vi "DCAM_example_multifunc_scmos_frame_acquisition.vi"() -> ()   [LabVIEW 2015]
uses:
  <vilib>/Utility/miscctls.llb/LVRectTypeDef.ctl
panel:
  out "Image":u16[][](graph)
  in  "Stop Button":bool
  in  "Acquire Frames Button":bool
  in  "Take Snapshot Button":bool
  in  "Preview Mode Button":bool
  out "Start Trigger Mode":string
  out "error out":errorcluster
  out "Plot Area Bounds":T1
  in  "Exposure":dbl min=0.0010036691729323308 max=10.000004210526315 step=1e-08
  in  "Scan Mode":dbl min=1.0 max=2.0 step=1.0
  in  "Binning":u16(ring) items=["1x1"=1, "2x2"=2, "4x4"=4]
  out "Exposure":dbl
  out "Scan Mode":dbl
  out "S Vert Width":i32
  out "S Horiz Width":i32
  out "S Vert Offset":i32
  out "S Horiz Offset":i32
  in  "Vertical Width":i32 min=4 max=2048 step=4
  in  "Vertical Offset":i32 min=0 max=0 step=4
  in  "Horizontal Width":i32 min=4 max=2048 step=4
  in  "Horizontal Offset":i32 min=0 max=0 step=4
  in  "Number of Frames":dbl
  out "Timeseries Save Path":path
  out "Snapshot Save Path":path
  out "Timeseries Base Filename":string
  out "Snapshot Base Filename":string
  in  "Timeseries Base Filename":string
  in  "Timeseries Save Path":path
  in  "Snapshot Base Filename":string
  in  "Save Snapshots":bool caption="Save Snapshot"
  in  "Snapshot Save Path":path
  in  "Start Trigger Mode":u32(ring)=1 items=["Internal"=1, "External Edge"=2, "External Level"=4, "Software"=32, "Fast Repetition"=64, "TDI"=128, "Trigger Start"=512, "Sync Readout"=1024]
  out "Model":string
  out "Camera ID":string
  out "Firmware":string
  out "DCAM Ver.":string
  out "Library Ver.":string
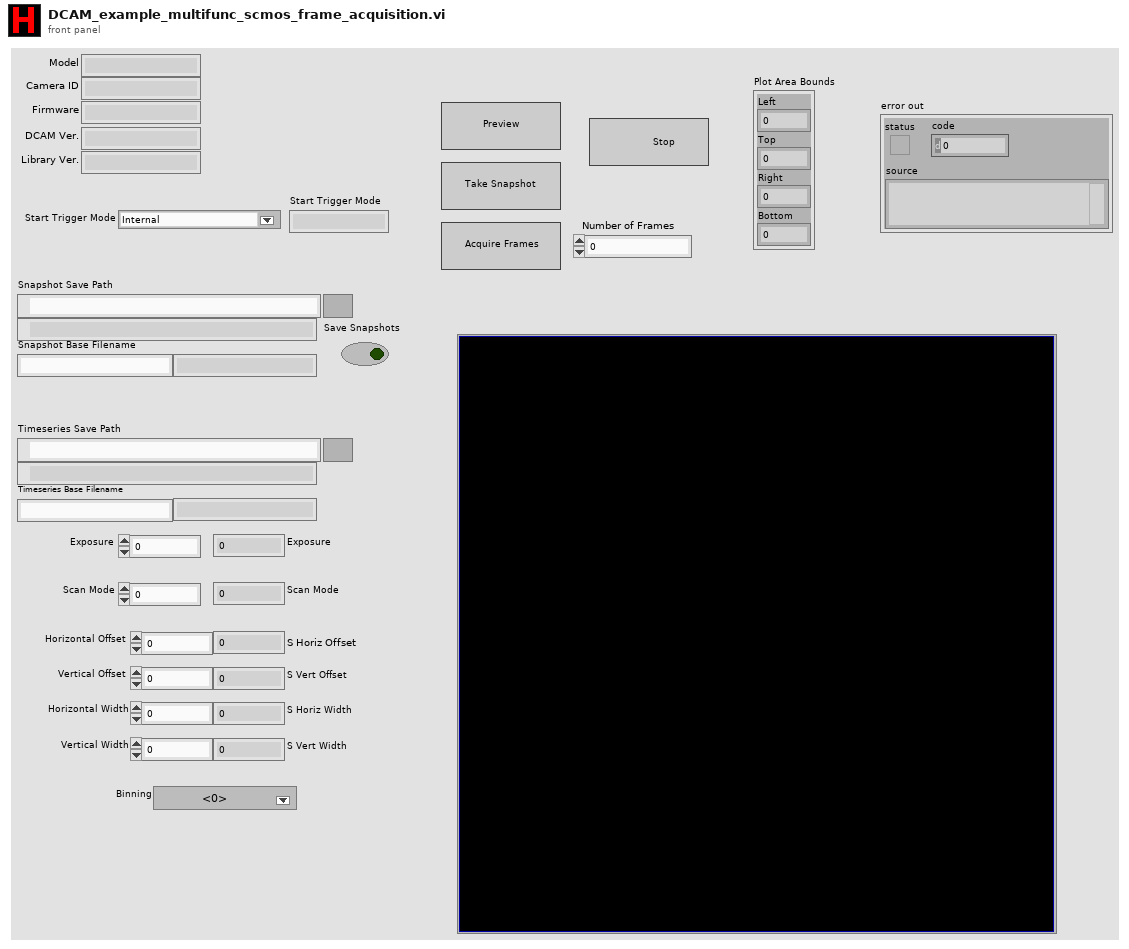
[diagram p1: front panel]
types:
  T1 = typedef "LVRectTypeDef.ctl" = cluster{"Left":i16, "Top":i16, "Right":i16, "Bottom":i16}
  T2 = cluster{"Capture Library":string, "DCAM-API":string}
  T3 = cluster{"Mode":u32, "Polarity":u16, "Times":u32, "Delay":dbl}
  T4 = cluster{"Mode":u32, "Polarity":u32, "Period":dbl, "Delay":dbl}
  T5 = cluster{"Model":string, "Camera ID":string, "Firmware":string}
  T6 = cluster{"Value":i32, "Minimum":i32, "Maximum":i32, "Increment":i32}
  T7 = cluster{"height":u32, "width":u32, "datatype":u32}
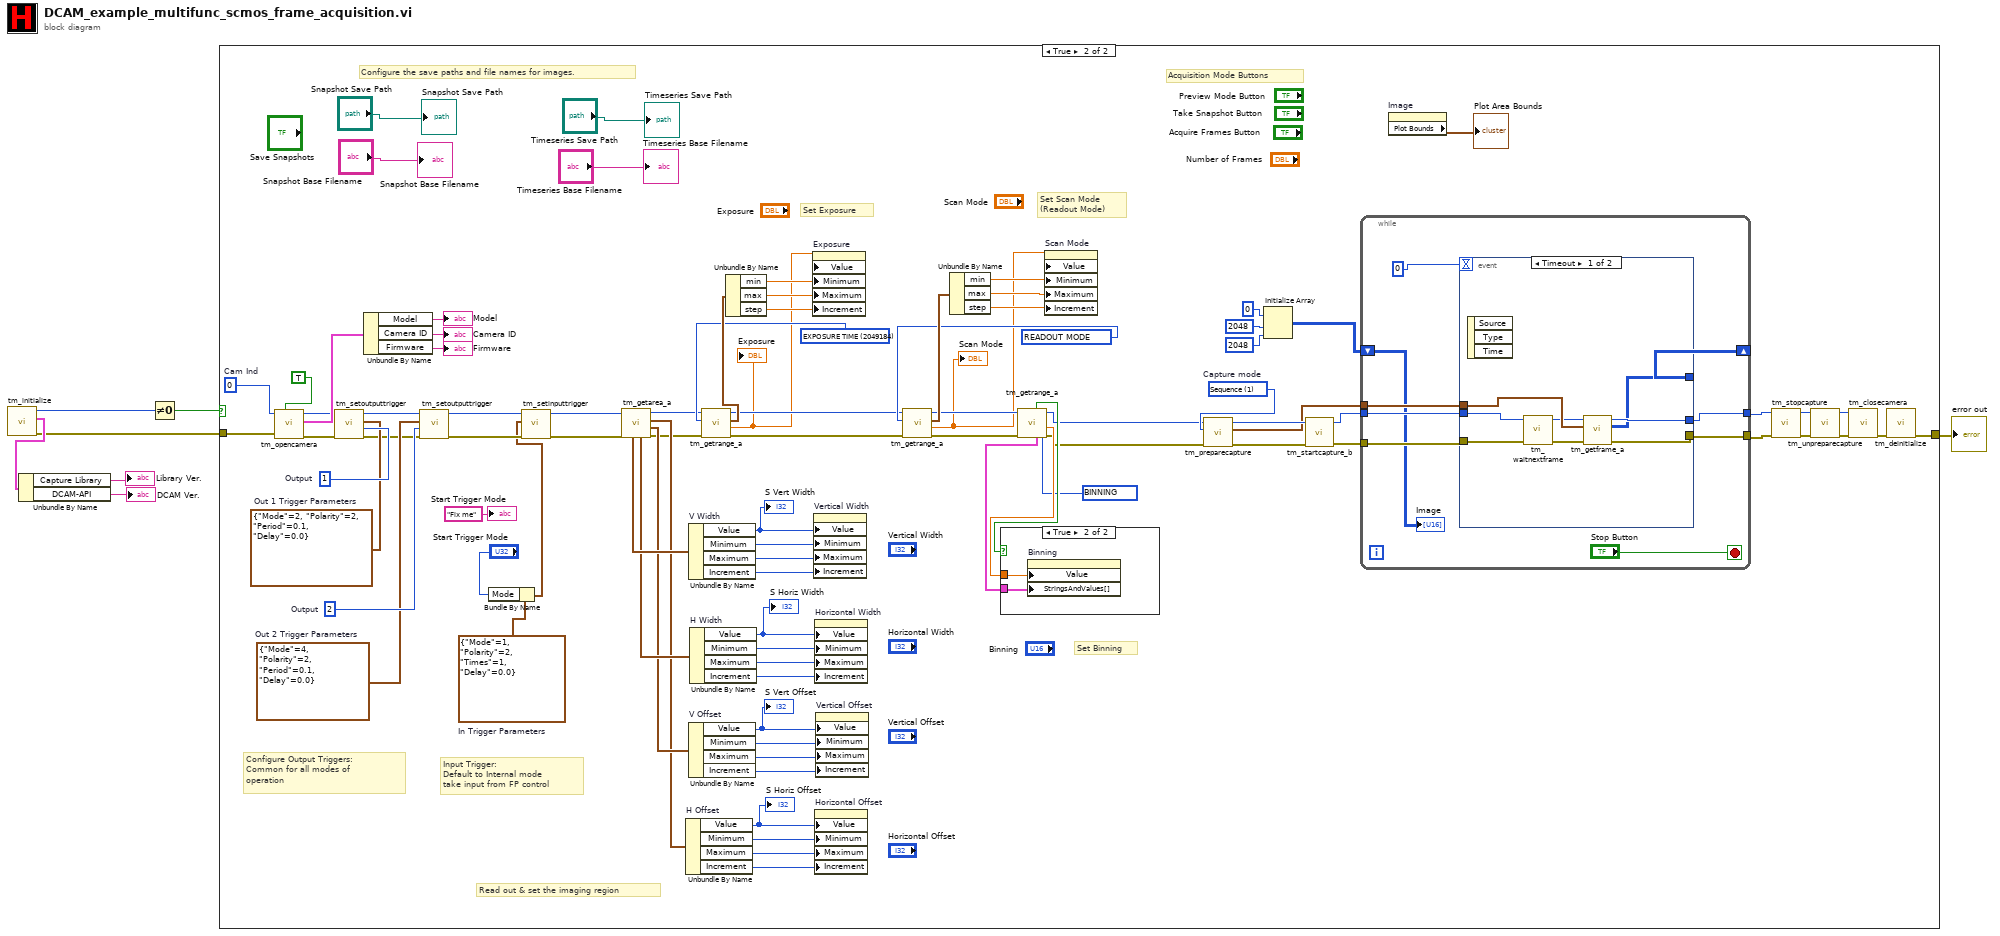
[diagram p0: block diagram]
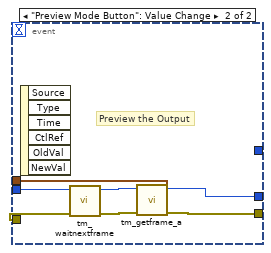
[diagram p3: hidden frame]
diagram:
  n1 = call <userlib>:"tm_initialize.vi"() -> ("error out"=w3:errorcluster, "Version Info"=w4:T2, "Number Of Cameras"=w7:u32)  [unwired: 8 in, 1 out]
  n2 = Unbundle By Name(w4) -> ("Capture Library"=→"Library Ver.":string, "DCAM-API"=→"DCAM Ver.":string)
  n3 = Not Equal To 0?(x=w7) -> (x != 0?=w2:bool)
  n4 = case shown="True" w2 {
    tunnel: w3 -> [w8 w85]
    tunnel: [w8 w37] -> w1
    frame False {
    }
    frame True {
      w20 = 1 items=["Snap", "Sequence"]  # Capture mode
      w47 = u32 2049184 items=["BINNING"=4215968, "BITS PER CHANNEL"=4342976, "ACTIVE VIEW INDEX"=4343136, "CCD MODE"=4212384, "SENSOR MODE"=4212128, "READOUT MODE"=4211872, "EXPOSURE TIME"=2049184, "CONTRAST GAIN"=3163312, "CONTRAST OFFSET"=3163328, "LIGHT MODE"=2114720, "SENSITIVITY"=2114992, "WHITE BALANCE"=3163568, "PHOTON IMAGING MODE"=2115200, "HIGH DYNAMIC RANGE MODE"=3163360, "TRIGGER SOURCE"=1066144, "TRIGGER ACTIVE"=1066160, "TRIGGER MODE"=1066400, "TRIGGER POLARITY"=1066416, "TRIGGER GLOBAL EXPOSURE"=2049680, "FIRST TRIGGER BEHAVIOR"=2049696, "TRIGGER TIMES"=1066448, "OUTPUT TRIGGER POLARITY"=1852592, "OUTPUT TRIGGER DELAY"=1852624, "OUTPUT TRIGGER PERIOD"=1852640, "TEMPERATURE"=2115232, "TEMPERATURE TARGET"=2115264, "SENSOR COOLER FAN"=2115296, "MECHANICAL SHUTTER"=2115488, "BACK FOCUS POSITION"=8422304, "FRAMEBUNDLE MODE"=4346784, "FRAMEBUNDLE NUMBER"=4346800, "LINEBUNDLE HEIGHT"=4212192, "TRIGGER CONNECTOR"=1066432, "IMAGE PIXEL TYPE"=4343296, "OUTPUT TRIGGER KIND"=1852656, "READOUT DIRECTION"=4211904, "CHANNEL SYNC"=1852352] ("Parameter")
      w48 = u32 4211872 items=["BINNING"=4215968, "BITS PER CHANNEL"=4342976, "ACTIVE VIEW INDEX"=4343136, "CCD MODE"=4212384, "SENSOR MODE"=4212128, "READOUT MODE"=4211872, "EXPOSURE TIME"=2049184, "CONTRAST GAIN"=3163312, "CONTRAST OFFSET"=3163328, "LIGHT MODE"=2114720, "SENSITIVITY"=2114992, "WHITE BALANCE"=3163568, "PHOTON IMAGING MODE"=2115200, "HIGH DYNAMIC RANGE MODE"=3163360, "TRIGGER SOURCE"=1066144, "TRIGGER ACTIVE"=1066160, "TRIGGER MODE"=1066400, "TRIGGER POLARITY"=1066416, "TRIGGER GLOBAL EXPOSURE"=2049680, "FIRST TRIGGER BEHAVIOR"=2049696, "TRIGGER TIMES"=1066448, "OUTPUT TRIGGER POLARITY"=1852592, "OUTPUT TRIGGER DELAY"=1852624, "OUTPUT TRIGGER PERIOD"=1852640, "TEMPERATURE"=2115232, "TEMPERATURE TARGET"=2115264, "SENSOR COOLER FAN"=2115296, "MECHANICAL SHUTTER"=2115488, "BACK FOCUS POSITION"=8422304, "FRAMEBUNDLE MODE"=4346784, "FRAMEBUNDLE NUMBER"=4346800, "LINEBUNDLE HEIGHT"=4212192, "TRIGGER CONNECTOR"=1066432, "IMAGE PIXEL TYPE"=4343296, "OUTPUT TRIGGER KIND"=1852656, "READOUT DIRECTION"=4211904, "CHANNEL SYNC"=1852352] ("Parameter")
      w49 = u32 4215968 items=["BINNING"=4215968, "BITS PER CHANNEL"=4342976, "ACTIVE VIEW INDEX"=4343136, "CCD MODE"=4212384, "SENSOR MODE"=4212128, "READOUT MODE"=4211872, "EXPOSURE TIME"=2049184, "CONTRAST GAIN"=3163312, "CONTRAST OFFSET"=3163328, "LIGHT MODE"=2114720, "SENSITIVITY"=2114992, "WHITE BALANCE"=3163568, "PHOTON IMAGING MODE"=2115200, "HIGH DYNAMIC RANGE MODE"=3163360, "TRIGGER SOURCE"=1066144, "TRIGGER ACTIVE"=1066160, "TRIGGER MODE"=1066400, "TRIGGER POLARITY"=1066416, "TRIGGER GLOBAL EXPOSURE"=2049680, "FIRST TRIGGER BEHAVIOR"=2049696, "TRIGGER TIMES"=1066448, "OUTPUT TRIGGER POLARITY"=1852592, "OUTPUT TRIGGER DELAY"=1852624, "OUTPUT TRIGGER PERIOD"=1852640, "TEMPERATURE"=2115232, "TEMPERATURE TARGET"=2115264, "SENSOR COOLER FAN"=2115296, "MECHANICAL SHUTTER"=2115488, "BACK FOCUS POSITION"=8422304, "FRAMEBUNDLE MODE"=4346784, "FRAMEBUNDLE NUMBER"=4346800, "LINEBUNDLE HEIGHT"=4212192, "TRIGGER CONNECTOR"=1066432, "IMAGE PIXEL TYPE"=4343296, "OUTPUT TRIGGER KIND"=1852656, "READOUT DIRECTION"=4211904, "CHANNEL SYNC"=1852352] ("Parameter")
      w80 = T3 {"Mode"=1, "Polarity"=2, "Times"=1, "Delay"=0.0}  # In Trigger Parameters
      w86 = T4 {"Mode"=4, "Polarity"=2, "Period"=0.1, "Delay"=0.0}  # Out 2 Trigger Parameters
      w87 = T4 {"Mode"=2, "Polarity"=2, "Period"=0.1, "Delay"=0.0}  # Out 1 Trigger Parameters
      w89 = 2  # Output
      w91 = 1  # Output
      w97 = 0  # Cam Ind
      # "Acquisition Mode Buttons"
      # "Configure the save paths and file names for images."
      # "Set Binning"
      # "Set Scan Mode \n(Readout Mode)"
      # "Set Exposure"
      # "Read out & set the imaging region"
      # "Input Trigger:\nDefault to Internal mode\ntake input from FP control"
      # "Configure Output Triggers: \nCommon for all modes of operation"
      n5 = call <userlib>:"tm_opencamera.vi"("Force Open"=TRUE, "error in (no error)"=w85, "Camera Index"=w97) -> ("error out"=w84:errorcluster, "Camera Details"=w96:T5, "Handle out"=w92:u32)  [unwired: 6 in]
      n6 = call <userlib>:"tm_setoutputtrigger.vi"("error in (no error)"=w84, "Index"=w91, "Parameters"=w87) -> ("error out"=w83:errorcluster, "Handle out"=w90:u32)  [unwired: 7 in]
      n7 = Unbundle By Name(w96) -> ("Model"=→"Model":string, "Camera ID"=→"Camera ID":string, "Firmware"=→"Firmware":string)
      n8 = call <userlib>:"tm_setoutputtrigger.vi"("error in (no error)"=w83, "Index"=w89, "Parameters"=w86, "Handle in"=w90) -> ("error out"=w82:errorcluster)  [unwired: 6 in, 1 out]
      n9 = Bundle By Name(cluster=w80, "Mode"="Start Trigger Mode") -> (w81:T3)
      n10 = call <userlib>:"tm_setinputtrigger.vi"("error in (no error)"=w82, "Parameters"=w81, "Handle in"=w92) -> ("error out"=w77:errorcluster, "Handle out"=w78:u32)  [unwired: 7 in]
      n11 = call <userlib>:"tm_getarea_a.vi"("error in (no error)"=w77, "Handle in"=w78) -> ("error out"=w46:errorcluster, "V Offset"=w74:T6, "H Offset"=w73:T6, "Handle out"=w45:u32, "H Width"=w75:T6, "V Width"=w76:T6)  [unwired: 4 in]
      n12 = Unbundle By Name "H Offset"(w73) -> ("Value"=w60:i32, "Minimum"=w59:i32, "Maximum"=w58:i32, "Increment"=w57:i32)
      "S Horiz Offset" <- w60
      n13 = Unbundle By Name "V Width"(w76) -> ("Value"=w72:i32, "Minimum"=w71:i32, "Maximum"=w70:i32, "Increment"=w69:i32)
      "S Vert Width" <- w72
      n14 = Unbundle By Name "V Offset"(w74) -> ("Value"=w64:i32, "Minimum"=w63:i32, "Maximum"=w62:i32, "Increment"=w61:i32)
      "S Vert Offset" <- w64
      n15 = Unbundle By Name "H Width"(w75) -> ("Value"=w68:i32, "Minimum"=w67:i32, "Maximum"=w66:i32, "Increment"=w65:i32)
      "S Horiz Width" <- w68
      n16 = call <userlib>:"tm_getrange_a.vi"("error in (no error)"=w46, "Parameter"=w47, "Handle in"=w45) -> ("error out"=w55:errorcluster, "default"=w31:dbl, "Range"=w56:cluster{"min":dbl, "max":dbl, "step":dbl}, "Handle out"=w44:u32)  [unwired: 2 in, 3 out]
      "Exposure" <- w31
      n17 = Unbundle By Name(w56) -> ("min"=w32:dbl, "max"=w33:dbl, "step"=w34:dbl)
      n18 = property on="Exposure" class="DigNum (strict)"("Value"=w31, "Minimum"=w32, "Maximum"=w33, "Increment"=w34) -> ()  [unwired: 2 in, 2 out]
      n19 = property on="Vertical Width" class="DigNum (strict)"("Value"=w72, "Minimum"=w71, "Maximum"=w70, "Increment"=w69) -> ()  [unwired: 2 in, 2 out]
      n20 = property on="Horizontal Width" class="DigNum (strict)"("Value"=w68, "Minimum"=w67, "Maximum"=w66, "Increment"=w65) -> ()  [unwired: 2 in, 2 out]
      n21 = property on="Horizontal Offset" class="DigNum (strict)"("Value"=w60, "Minimum"=w59, "Maximum"=w58, "Increment"=w57) -> ()  [unwired: 2 in, 2 out]
      n22 = property on="Vertical Offset" class="DigNum (strict)"("Value"=w64, "Minimum"=w63, "Maximum"=w62, "Increment"=w61) -> ()  [unwired: 2 in, 2 out]
      n23 = call <userlib>:"tm_getrange_a.vi"("error in (no error)"=w55, "Parameter"=w48, "Handle in"=w44) -> ("error out"=w53:errorcluster, "default"=w27:dbl, "Range"=w54:cluster{"min":dbl, "max":dbl, "step":dbl}, "Handle out"=w43:u32)  [unwired: 2 in, 3 out]
      "Scan Mode" <- w27
      n24 = Unbundle By Name(w54) -> ("min"=w28:dbl, "max"=w29:dbl, "step"=w30:dbl)
      n25 = call <userlib>:"tm_getrange_a.vi"("error in (no error)"=w53, "Parameter"=w49, "Handle in"=w43) -> ("error out"=w18:errorcluster, "default"=w51:dbl, "Handle out"=w19:u32, "Value Names"=w50:cluster{"Name":string, "Value":dbl}[], "Writable"=w52:bool)  [unwired: 2 in, 2 out]
      n26 = case shown="True" w52 {
        tunnel: w50 -> [_ w122]
        tunnel: w51 -> [_ w123]
        frame False {
        }
        frame True {
          n27 = property on="Binning" class="Ring (strict)"("Value"=w123, "StringsAndValues[]"=w122) -> ()  [unwired: 2 in, 2 out]
        }
      }
      n28 = property on="Scan Mode" class="DigNum (strict)"("Value"=w27, "Minimum"=w28, "Maximum"=w29, "Increment"=w30) -> ()  [unwired: 2 in, 2 out]
      n29 = call <userlib>:"tm_preparecapture.vi"("error in (no error)"=w18, "Capture mode"=w20, "Handle in"=w19) -> ("error out"=w15:errorcluster, "Buffer Info"=w14:T7, "Handle out"=w17:u32)  [unwired: 5 in, 1 out]
      n30 = Initialize Array(u16 0 ("element"), 2048 ("dimension size"), 2048 ("dimension size")) -> (w11:u16[][])
      n31 = call <userlib>:"tm_startcapture_b.vi"("error in (no error)"=w15, "Handle in"=w17) -> ("error out"=w16:errorcluster, "Handle out"=w13:u32)  [unwired: 8 in]
      n32 = while {
        tunnel: w13 -> [w104]
        tunnel: [w105] -> w35
        tunnel: [w106] -> w36
        tunnel: w16 -> [w102]
        tunnel: w14 -> [w103]
        shift-right: [w99] -> _
        shift-left: w11 -> [w98]
        stop <- "Stop Button" stop-if-true
        n33 = event shown="[0] Timeout" {
          selector: _ -> [_ _]
          dyn-events: _ -> [_ _]
          timeout: 0 -> [_ _]
          tunnel: [w110 w121] -> w106
          tunnel: [w109 w120] -> w105
          tunnel: w104 -> [w113 w119]
          tunnel: w103 -> [w114 w118]
          tunnel: w102 -> [w112 w117]
          tunnel: [w108 _] -> w99
          event Timeout {
            n34 = event-data() -> ()  [unwired: 1 in, 3 out]
            n35 = call <userlib>:"tm_waitnextframe.vi"("error in (no error)"=w112, "Handle in"=w113) -> ("error out"=w111:errorcluster, "Handle out"=w107:u32)  [unwired: 6 in, 2 out]
            n36 = call <userlib>:"tm_getframe_a.vi"("error in (no error)"=w111, "Buffer Info"=w114, "Handle in"=w107) -> ("error out"=w110:errorcluster, "Data 16"=w108:u16[][], "Handle out"=w109:u32)  [unwired: 4 in, 2 out]
          }
          event "Preview Mode Button": Value Change {
            # "Preview the Output"
            n37 = event-data() -> ()  [unwired: 1 in, 6 out]
            n38 = call <userlib>:"tm_waitnextframe.vi"("error in (no error)"=w117, "Handle in"=w119) -> ("error out"=w115:errorcluster, "Handle out"=w116:u32)  [unwired: 6 in, 2 out]
            n39 = call <userlib>:"tm_getframe_a.vi"("error in (no error)"=w115, "Buffer Info"=w118, "Handle in"=w116) -> ("error out"=w121:errorcluster, "Handle out"=w120:u32)  [unwired: 4 in, 3 out]
          }
        }
        "Image" <- w98
      }
      n40 = property on="Image" class="IntGraph (strict)"() -> ("Plot Bounds"=→"Plot Area Bounds":T1)  [unwired: 2 in, 2 out]
      n41 = call <userlib>:"tm_stopcapture.vi"("error in (no error)"=w36, "Handle in"=w35) -> ("error out"=w41:errorcluster, "Handle out"=w40:u32)  [unwired: 8 in]
      n42 = call <userlib>:"tm_unpreparecapture.vi"("error in (no error)"=w41, "Handle in"=w40) -> ("error out"=w42:errorcluster, "Handle out"=w39:u32)  [unwired: 8 in]
      n43 = call <userlib>:"tm_closecamera.vi"("error in (no error)"=w42, "Handle in"=w39) -> ("error out"=w38:errorcluster)  [unwired: 9 in]
      n44 = call <userlib>:"tm_deinitialize.vi"("error in (no error)"=w38) -> ("error out"=w37:errorcluster)  [unwired: 10 in]
      "Timeseries Base Filename" <- "Timeseries Base Filename"
      "Timeseries Save Path" <- "Timeseries Save Path"
      "Snapshot Base Filename" <- "Snapshot Base Filename"
      "Snapshot Save Path" <- "Snapshot Save Path"
      "Start Trigger Mode" <- "Fix me"
    }
  }
  "error out" <- w1
